vi "SetTS.vi"(8 "Acquisition Settings":T1, 11 "timeslice":T3) -> ()   [LabVIEW 2014]
uses:
  Timeslice.ctl
  DAQSettings.ctl
  TriggerMode.ctl
panel:
  out "outputClockData":u32[](array[numeric])
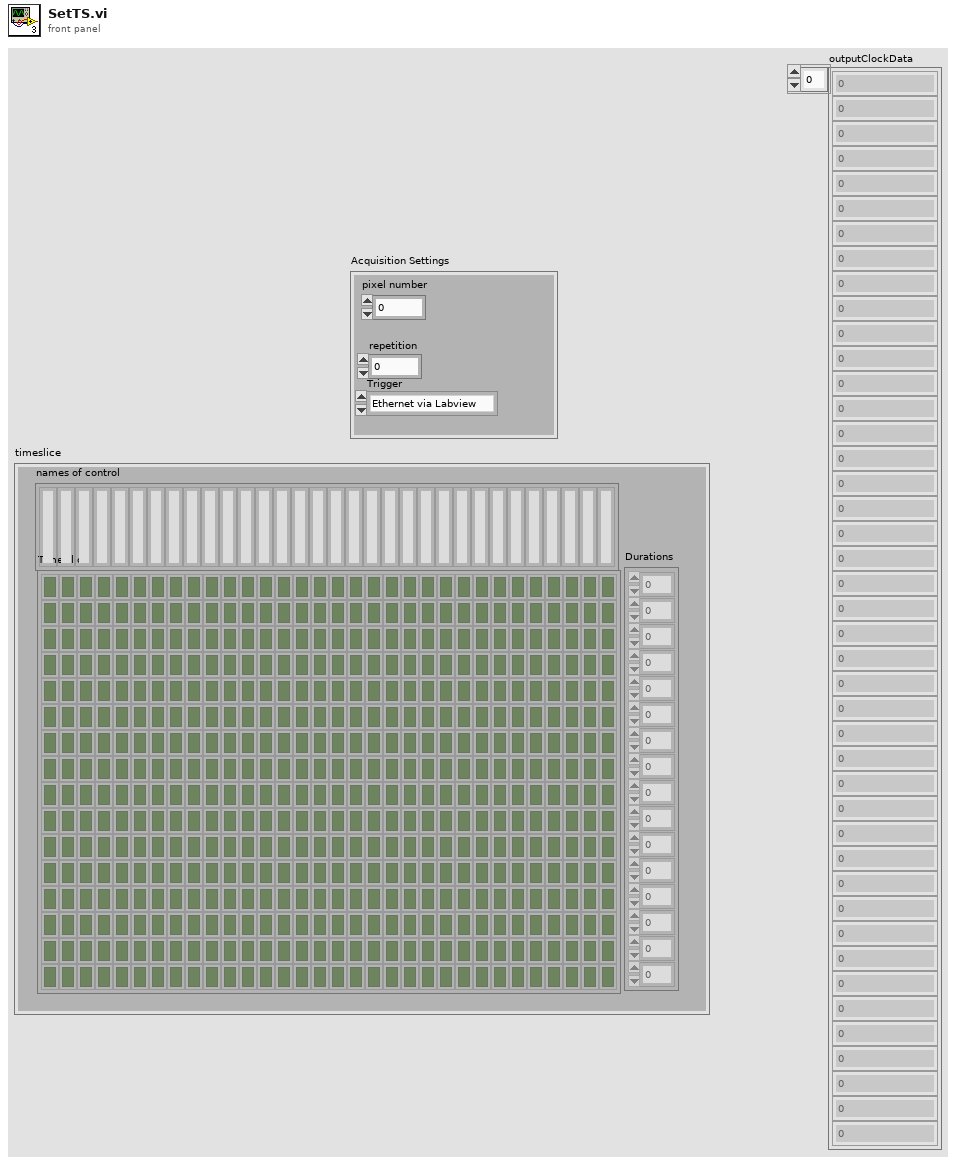
[diagram p1: front panel]
types:
  T1 = typedef "DAQSettings.ctl" = cluster{"pixel number":u32, "repetition":u32, "Trigger":T2}
  T2 = typedef "TriggerMode.ctl" = enum16{"Ethernet via Labview", "SMA (1.8V)"}
  T3 = typedef "Timeslice.ctl" = cluster{"Time slice":bool[][], "Durations":dbl[], "names of control":string[]}
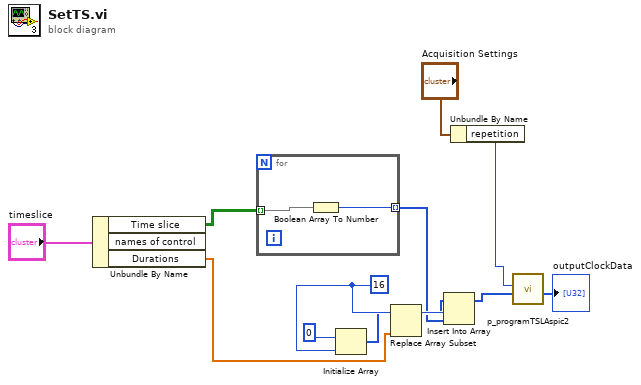
[diagram p0: block diagram]
diagram:
  w12 = 16 ("index")
  n1 = Unbundle By Name("timeslice") -> ("Time slice"=w7:bool[][], "Durations"=w4:dbl[])  [unwired: 1 out]
  n2 = for {
    tunnel: w7 -> [w14] mode=indexing
    tunnel: [w13] -> w6 mode=indexing
    n3 = Boolean Array To Number(Boolean array=w14) -> (number=w13:u32)
  }
  n4 = Initialize Array(u32 0 ("element"), w12) -> (w10:u32[])
  n5 = Replace Array Subset(array=w10, new element=w4) -> (w11:u32[])  [unwired: 1 in]
  n6 = Insert Into Array(array=w11, index=w12, new element=w6) -> (w2:u32[])
  n7 = Unbundle By Name("Acquisition Settings") -> ("repetition"=w3:u32)
  n8 = call "p_programTSLAspic2.vi"("clockdata 2"=w2, "repetitions"=w3) -> ("outputClockData"=→"outputClockData":u32[])  [unwired: 8 in, 1 out]
